vi "prep.vi"(8 "error in (no error)":errorcluster, 9 "Coordinate System":enum16{"Cartesian", "Cylindrical", "Spherical"}(ring), 10 "Plot processed data In":T1 caption="Data In", 11 "Parametric in":refnum<class "Parametric.lvclass">) -> (0 "error out":errorcluster, 2 "Plot Processed Data Out":T1 caption="Data Out", 3 "Parametric out":refnum<class "Parametric.lvclass">)   [LabVIEW 2020, in "Parametric.lvclass"]
uses:
  <vilib>/Native 3D Graph/classes/Parametric/Parametric.lvclass
  <vilib>/Native 3D Graph/xcontrol/Processed Data.ctl
  <vilib>/Native 3D Graph/typedefs/plot_rep_array.ctl
  <vilib>/Native 3D Graph/typedefs/plot_rep.ctl
  <vilib>/Native 3D Graph/typedefs/range_cluster.ctl
  <vilib>/Native 3D Graph/typedefs/min_max.ctl
  <vilib>/Native 3D Graph/typedefs/plot_rep_mesh_data.ctl
  <vilib>/Native 3D Graph/classes/Parametric/Parametric.lvclass/Parametric.ctl
  <vilib>/Analysis/coordinate.llb/3D Coordinate Conversion (Scalar).vi
  <vilib>/Native 3D Graph/classes/Base Datatype.lvclass
  <vilib>/Native 3D Graph/xcontrol/3DPC_SurfacePlot.xctl
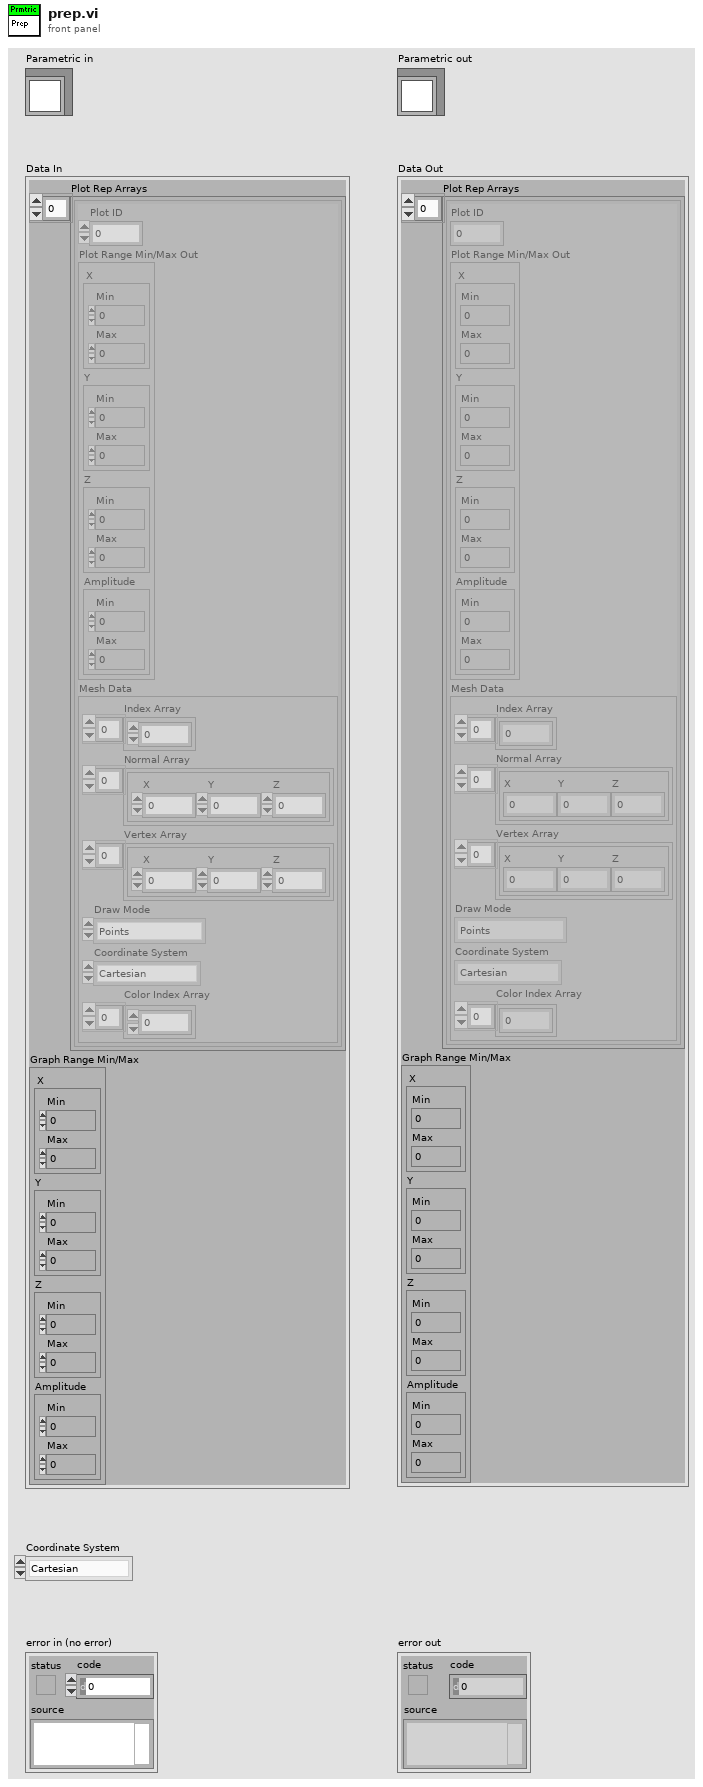
[diagram p1: front panel]
types:
  T1 = typedef "Processed Data.ctl" = cluster{"Plot Rep Arrays":T2, "Graph Range Min/Max":T4}
  T2 = typedef "3DPC_SurfacePlot.xctl/plot_rep_array.ctl" = T3[]
  T3 = typedef "3DPC_SurfacePlot.xctl/plot_rep.ctl" = cluster{"Plot ID":i32, "Plot Range Min/Max Out":T4, "Mesh Data":T6}
  T4 = typedef "3DPC_SurfacePlot.xctl/range_cluster.ctl" = cluster{"X":T5, "Y":T5, "Z":T5, "Amplitude":T5}
  T5 = typedef "3DPC_SurfacePlot.xctl/min_max.ctl" = cluster{"Min":sgl, "Max":sgl}
  T6 = typedef "3DPC_SurfacePlot.xctl/plot_rep_mesh_data.ctl" = cluster{"Index Array":u32[], "Normal Array":cluster{"X":sgl, "Y":sgl, "Z":sgl}[], "Vertex Array":cluster{"X":sgl, "Y":sgl, "Z":sgl}[], "Draw Mode":enum16{"Points", "Lines", "Line Strip", "Line Loop", "Triangles", "Triangle Strip", "Triangle Fan", "Quads", "Quad Strip", "Polygon"}, "Coordinate System":enum16{"Cartesian", "Cylindrical", "Spherical"}, "Color Index Array":i32[]}
  T7 = enum16{"Points", "Lines", "Line Strip", "Line Loop", "Triangles", "Triangle Strip", "Triangle Fan", "Quads", "Quad Strip", "Polygon"}
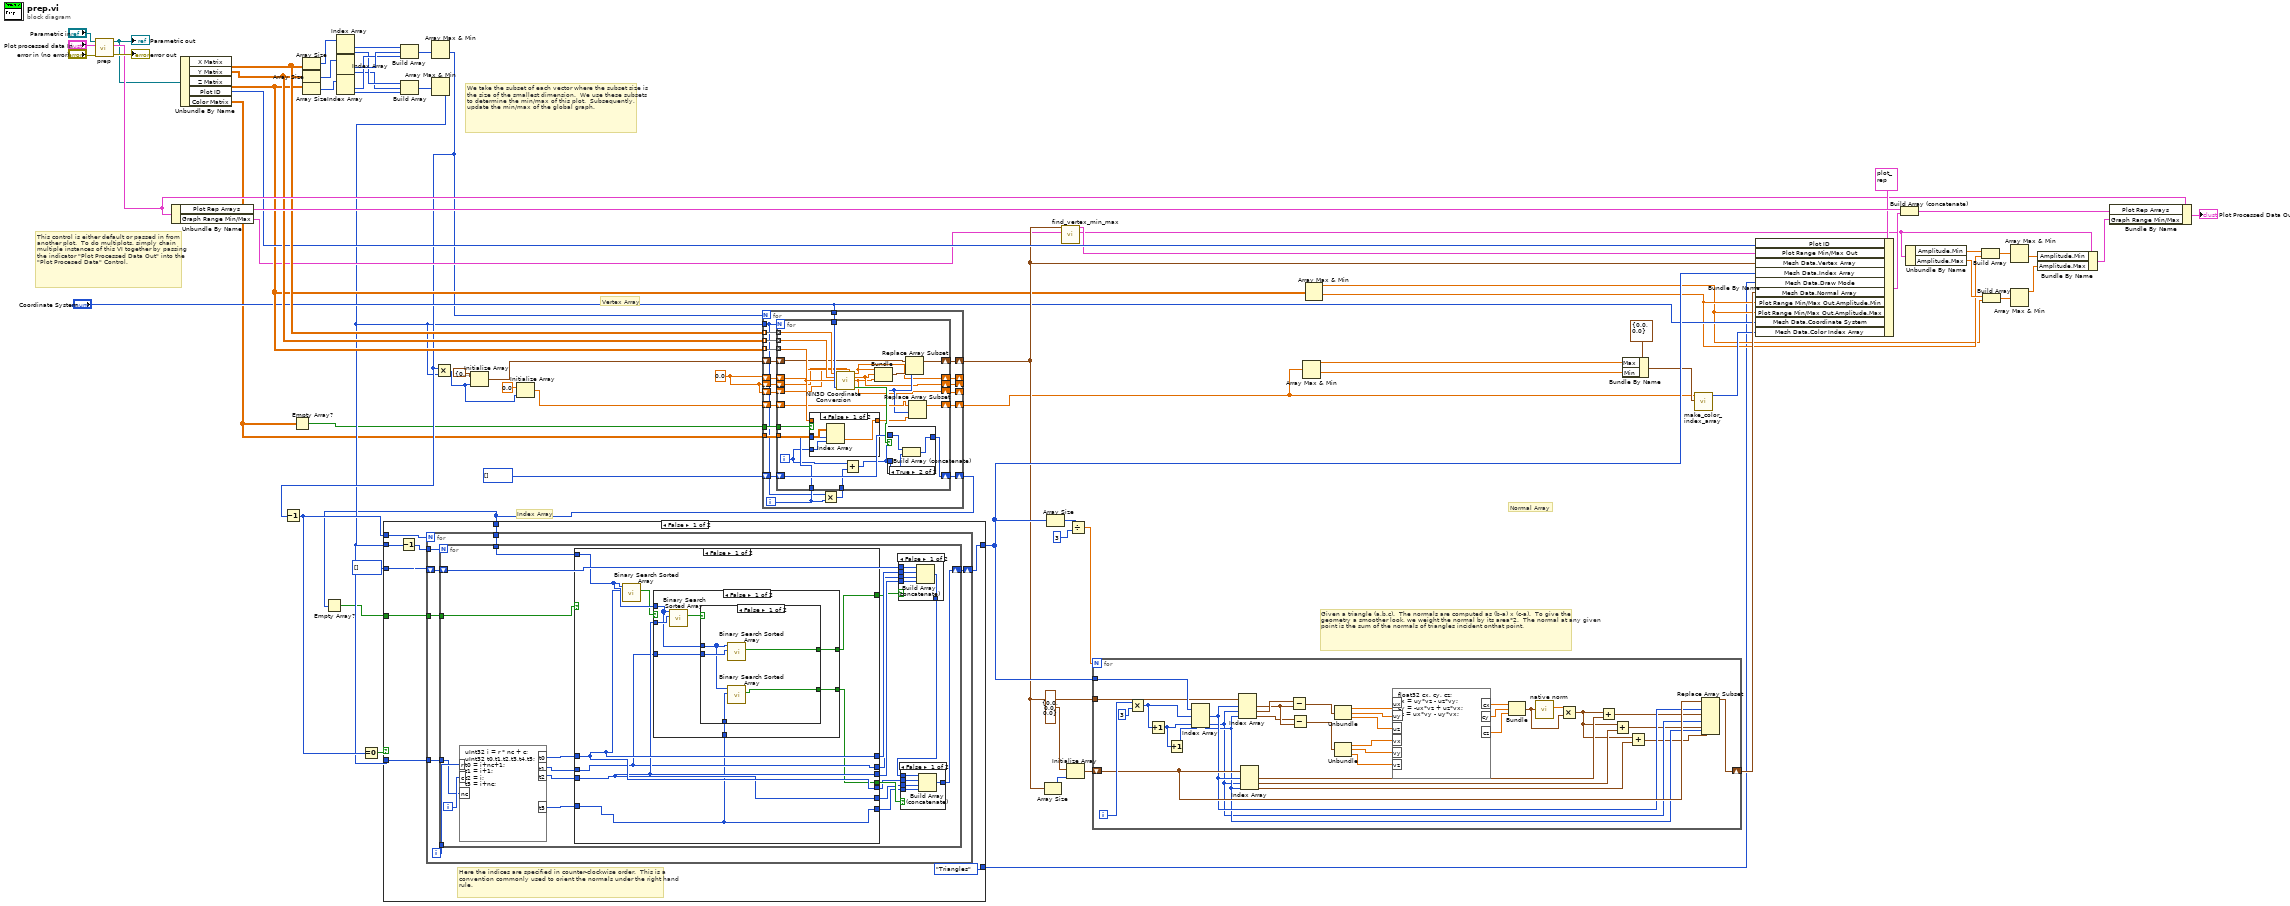
[diagram p0: block diagram]
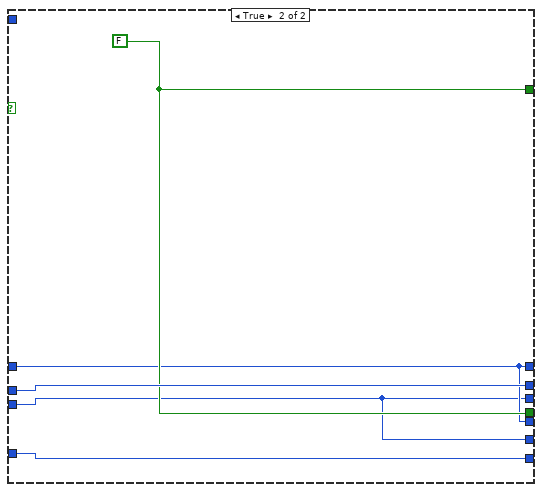
[diagram p6: hidden frame]
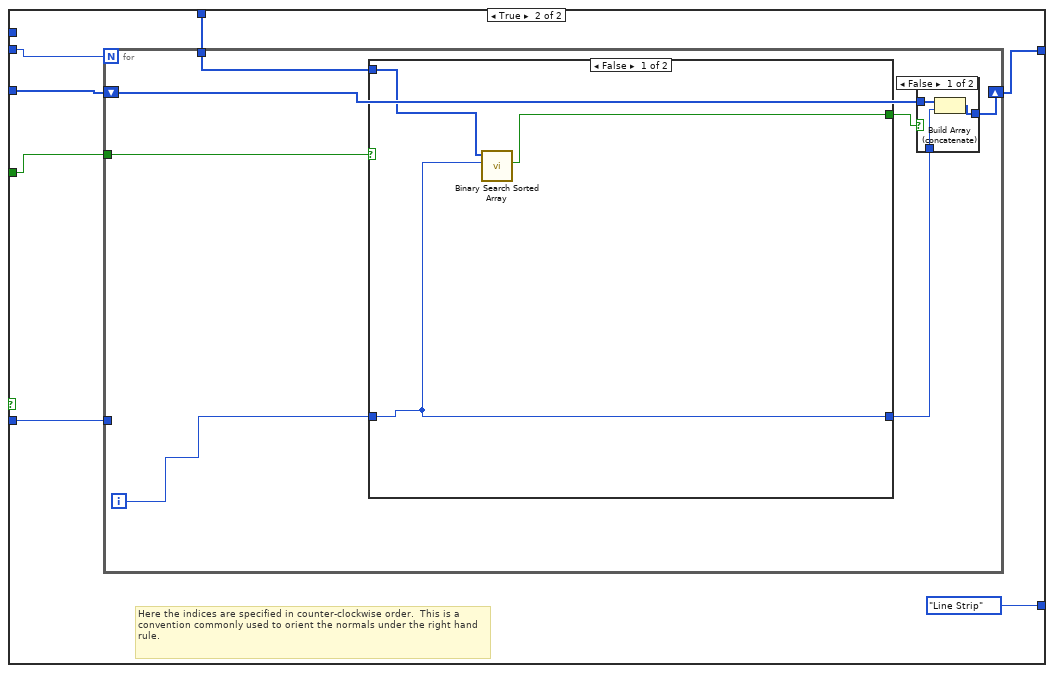
[diagram p7: hidden frame]
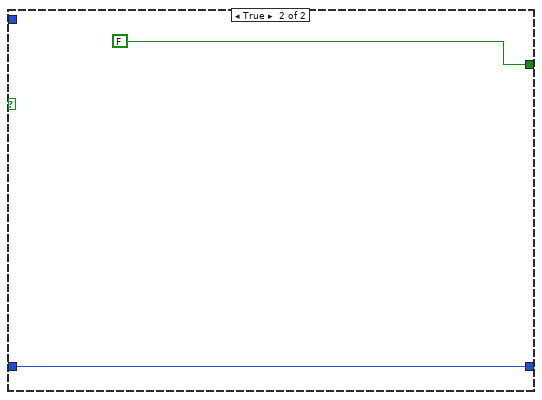
[diagram p9: hidden frame]
diagram:
  w7 = sgl 0.0
  # "Given a triangle (a,b,c).  The normals are computed as (b-a) x (c-a).  To give the geometry a smoother look, we weight the normal by its area*2.  The normal at any given point is the sum of the normals of triangles incident onthat point."
  # "Normal Array"
  # "Index Array"
  # "We take the subset of each vector where the subset size is the size of the smallest dimension.  We use these subsets to determine the min/max of this plot.  Subsequently, update the min/max of the global graph."
  # "This control is either default or passed in from another plot.  To do multiplots, simply chain multiple instances of this VI together by passing the indicator \"Plot Processed Data Out\" into the \"Plot Procesed Data\" Control."
  # "Vertex Array"
  n1 = call-parent "prep.vi"("error in (no error)"="error in (no error)", "Plot processed data In"="Plot processed data In", "Base Datatype in"="Parametric in") -> ("error out"=→"error out":errorcluster, "Plot processed Data Out"=w42:T1, "Base Datatype out"=w41:refnum<class "Parametric.lvclass">)  [unwired: 1 in, 5 out]
  "Parametric out" <- w41
  n2 = Unbundle By Name(w42) -> ("Plot Rep Arrays"=w66:T2, "Graph Range Min/Max"=w34:T4)
  n3 = Unbundle By Name(w41) -> ("X Matrix"=w40:sgl[][], "Y Matrix"=w39:sgl[][], "Z Matrix"=w35:sgl[][], "Plot ID"=w38:i32, "Color Matrix"=w4:sgl[][])
  n4 = Empty Array?(array=w4) -> (empty?=w3:bool)
  n5 = Array Size(array=w40) -> (size(s)=w62:i32[])
  n6 = Array Size(array=w39) -> (size(s)=w61:i32[])
  n7 = Array Size(array=w35) -> (size(s)=w60:i32[])
  n8 = Index Array(array=w62) -> (element #1=w59:i32, element #2=w56:i32)  [unwired: 2 in]
  n9 = Index Array(array=w61) -> (element #1=w58:i32, element #2=w55:i32)  [unwired: 2 in]
  n10 = Index Array(array=w60) -> (element #1=w57:i32, element #2=w54:i32)  [unwired: 2 in]
  n11 = Build Array(w59, w58, w57) -> (w53:i32[])
  n12 = Build Array(w56, w55, w54) -> (w52:i32[])
  n13 = Array Max & Min(array=w53) -> (min value=w14:i32)  [unwired: 3 out]
  n14 = Decrement(x=w14) -> (x-1=w17:i32)
  n15 = Equal To 0?(x=w17) -> (x = 0?=w16:bool)
  n16 = Array Max & Min(array=w52) -> (min value=w13:i32)  [unwired: 3 out]
  n17 = Multiply(x=w14, y=w13) -> (x*y=w9:i32)
  n18 = Initialize Array(cluster{"X":sgl, "Y":sgl, "Z":sgl} {"X"=0.0, "Y"=0.0, "Z"=0.0} ("3D Point"), w9) -> (w11:cluster{"X":sgl, "Y":sgl, "Z":sgl}[])
  n19 = Initialize Array(sgl 0.0, w9) -> (w8:sgl[])
  n20 = for {
    N: w14 -> [_]
    tunnel: w40 -> [w92] mode=indexing
    tunnel: w39 -> [w91] mode=indexing
    tunnel: w35 -> [w90] mode=indexing
    tunnel: w13 -> [w79]
    shift-right: [w88] -> w37
    shift-left: w11 -> [w89]
    tunnel: "Coordinate System" -> [w87]
    shift-right: [w85] -> w20
    shift-left: w8 -> [w86]
    tunnel: w3 -> [w84]
    tunnel: w4 -> [w83]
    shift-right: [w81] -> w6
    shift-left: u32[] [] -> [w82]
    shift-right: [w74] -> _
    shift-left: w7 -> [w77]
    shift-right: [w73] -> _
    shift-left: w7 -> [w76]
    shift-right: [w72] -> _
    shift-left: w7 -> [w75]
    i -> [w80]
    n21 = Multiply(x=w79, y=w80) -> (x*y=w78:i32)
    n22 = for {
      N: w79 -> [_]
      shift-right: [w104] -> w88
      shift-left: w89 -> [w105]
      tunnel: w92 -> [w115] mode=indexing
      tunnel: w91 -> [w116] mode=indexing
      tunnel: w90 -> [w113] mode=indexing
      tunnel: w87 -> [w117]
      shift-right: [w101] -> w85
      shift-left: w86 -> [w102]
      tunnel: w84 -> [w114]
      tunnel: w83 -> [w112]
      tunnel: w80 -> [w108]
      shift-right: [w109] -> w81
      shift-left: w82 -> [w110]
      tunnel: w78 -> [w107]
      shift-right: [w95] -> w74
      shift-left: w77 -> [w98]
      shift-right: [w94] -> w73
      shift-left: w76 -> [w97]
      shift-right: [w93] -> w72
      shift-left: w75 -> [w96]
      i -> [w106]
      n23 = case shown="False" w114 {
        tunnel: w113 -> [_ w126]
        tunnel: [w122 w126] -> w99
        tunnel: w112 -> [w125 _]
        tunnel: w108 -> [w124 _]
        tunnel: w106 -> [w123 _]
        frame False {
          n24 = Index Array(array=w125, index (row)=w124, index (col)=w123) -> (element=w122:sgl)
        }
        frame True {
        }
      }
      n25 = call <vilib>:"NIN3D Coordinate Conversion.vi"("X"=w115, "Z_prev"=w96, "Y_prev"=w97, "X_prev"=w98, "Y"=w116, "Z"=w113, "Coordinate System"=w117) -> ("X out"=w95:sgl, "Y out"=w94:sgl, "Z out"=w93:sgl, "NaN?"=w111:bool)  [unwired: 5 in]
      n26 = Add(x=w106, y=w107) -> (x+y=w100:i32)
      n27 = Bundle("X out"=w95, "Y out"=w94, "Z out"=w93) -> (w103:cluster{"X out":sgl, "Y out":sgl, "Z out":sgl})  [unwired: 1 out]
      n28 = case shown="True" w111 {
        tunnel: w110 -> [w118 w121]
        tunnel: [w118 w120] -> w109
        tunnel: w100 -> [_ w119]
        frame False {
        }
        frame True {
          n29 = Build Array (concatenate)(w121, w119) -> (w120:u32[])
        }
      }
      n30 = Replace Array Subset(array=w105, new element=w103, index=w100) -> (w104:cluster{"X":sgl, "Y":sgl, "Z":sgl}[])
      n31 = Replace Array Subset(array=w102, new element=w99, index=w100) -> (w101:sgl[])
    }
  }
  n32 = Empty Array?(array=w6) -> (empty?=w5:bool)
  n33 = case shown="False" w16 {
    tunnel: u32[] [] ("Indices") -> [w127 w208]
    tunnel: w13 -> [w135 w207]
    tunnel: [w134 w206] -> w44
    tunnel: w17 -> [w133 _]
    tunnel: w6 -> [w132 w205]
    tunnel: w13 -> [w131 w204]
    tunnel: [T7."Triangles" ("Mesh Data.Draw Mode") T7."Line Strip" ("Mesh Data.Draw Mode")] -> w2
    tunnel: w5 -> [w128 w202]
    frame False {
      # "Here the indices are specified in counter-clockwise order.  This is a convention commonly used to orient the normals under the right hand rule."
      n34 = Decrement(x=w131) -> (x-1=w130:i32)
      n35 = for {
        N: w133 -> [_]
        shift-right: [w138] -> w134
        shift-left: w127 -> [w142]
        tunnel: w130 -> [w140]
        tunnel: w135 -> [w139]
        tunnel: w132 -> [w137]
        tunnel: w128 -> [w136]
        i -> [w141]
        n36 = for {
          N: w140 -> [_]
          tunnel: w141 -> [w161]
          tunnel: w139 -> [w159]
          shift-right: [w147] -> w138
          shift-left: w142 -> [w162]
          tunnel: w137 -> [w154]
          tunnel: w136 -> [w143]
          i -> [w160]
          n37 = formula code="uInt32 i = r * nc + c; \nuInt32 t0,t1,t2,t3,t4,t5;\nt0 = i+nc+1; \nt1 = i+1; \nt2 = i; \nt5 = i+nc;"("r"=w161, "nc"=w159, "c"=w160) -> ("t0"=w158:u32, "t1"=w157:u32, "t2"=w156:u32, "t5"=w155:u32)
          n38 = case shown="False" w143 {
            tunnel: w154 -> [w182 _]
            tunnel: w158 -> [w181 w198]
            tunnel: [w181 w198] -> w153
            tunnel: w157 -> [w177 w201]
            tunnel: [w177 w201] -> w152
            tunnel: w156 -> [w178 w197]
            tunnel: [w178 w197] -> w151
            tunnel: [w181 w198] -> w146
            tunnel: [w178 w197] -> w145
            tunnel: w155 -> [w176 w200]
            tunnel: [w176 w200] -> w144
            tunnel: [w180 w199] -> w150
            tunnel: [w175 w199] -> w149
            frame False {
              n39 = call <vilib>:"Binary Search Sorted Array.vi"("Element"=w181, "Sorted Array"=w182) -> ("Found?"=w179:bool)  [unwired: 9 in]
              n40 = case shown="False" w179 {
                selector: w179 -> [_ w196]
                tunnel: w182 -> [w187 _]
                tunnel: w178 -> [w189 _]
                tunnel: [w186 w196] -> w180
                tunnel: w177 -> [w185 _]
                tunnel: w176 -> [w184 _]
                tunnel: [w183 w196] -> w175
                frame False {
                  n41 = call <vilib>:"Binary Search Sorted Array.vi"("Element"=w189, "Sorted Array"=w187) -> ("Found?"=w188:bool)  [unwired: 9 in]
                  n42 = case shown="False" w188 {
                    selector: w188 -> [_ w195]
                    tunnel: w187 -> [w191 _]
                    tunnel: w185 -> [w194 _]
                    tunnel: [w193 w195] -> w186
                    tunnel: w184 -> [w192 _]
                    tunnel: [w190 w195] -> w183
                    frame False {
                      n43 = call <vilib>:"Binary Search Sorted Array.vi"("Element"=w194, "Sorted Array"=w191) -> ("Found?"=w193:bool)  [unwired: 9 in]
                      n44 = call <vilib>:"Binary Search Sorted Array.vi"("Element"=w192, "Sorted Array"=w191) -> ("Found?"=w190:bool)  [unwired: 9 in]
                    }
                    frame True {
                    }
                  }
                }
                frame True {
                }
              }
            }
            frame True {
              w199 = FALSE
            }
          }
          n45 = case shown="False" w150 {
            tunnel: w162 -> [w173 w174]
            tunnel: w153 -> [w172 _]
            tunnel: w152 -> [w171 _]
            tunnel: w151 -> [w170 _]
            tunnel: [w169 w174] -> w148
            frame False {
              n46 = Build Array (concatenate)(w173, w172, w171, w170) -> (w169:u32[])
            }
            frame True {
            }
          }
          n47 = case shown="False" w149 {
            tunnel: w148 -> [w167 w168]
            tunnel: [w166 w168] -> w147
            tunnel: w146 -> [w165 _]
            tunnel: w145 -> [w164 _]
            tunnel: w144 -> [w163 _]
            frame False {
              n48 = Build Array (concatenate)(w167, w165, w164, w163) -> (w166:u32[])
            }
            frame True {
            }
          }
        }
      }
    }
    frame True {
      # "Here the indices are specified in counter-clockwise order.  This is a convention commonly used to orient the normals under the right hand rule."
      n49 = for {
        N: w204 -> [_]
        tunnel: w207 -> [_]
        shift-right: [w214] -> w206
        shift-left: w208 -> [w215]
        tunnel: w205 -> [w213]
        tunnel: w202 -> [w209]
        i -> [w210]
        n50 = case shown="False" w209 {
          tunnel: w213 -> [w222 _]
          tunnel: w210 -> [w221 w223]
          tunnel: [w220 FALSE] -> w212
          tunnel: [w221 w223] -> w211
          frame False {
            n51 = call <vilib>:"Binary Search Sorted Array.vi"("Element"=w221, "Sorted Array"=w222) -> ("Found?"=w220:bool)  [unwired: 9 in]
          }
          frame True {
          }
        }
        n52 = case shown="False" w212 {
          tunnel: w215 -> [w218 w219]
          tunnel: [w217 w219] -> w214
          tunnel: w211 -> [w216 _]
          frame False {
            n53 = Build Array (concatenate)(w218, w216) -> (w217:u32[])
          }
          frame True {
          }
        }
      }
    }
  }
  n54 = Array Size(array=w37) -> (size(s)=w50:i32)
  n55 = Array Size(array=w44) -> (size(s)=w46:i32)
  n56 = call <vilib>:"find_vertex_min_max.vi"("Total Range Min/Max"=w34, "Vertex Array"=w37) -> ("Total Range Out"=w25:T4, "This Range Min/Max Out"=w36:T4)  [unwired: 8 out]
  n57 = Initialize Array(cluster{"X":sgl, "Y":sgl, "Z":sgl} {"X"=0.0, "Y"=0.0, "Z"=0.0} ("3D Point"), w50) -> (w49:cluster{"X":sgl, "Y":sgl, "Z":sgl}[])
  n58 = Divide(x=w46, y=3) -> (x/y=w47:dbl)
  n59 = for {
    N: w47 -> [_]
    shift-right: [w251] -> w43
    shift-left: w49 -> [w254]
    tunnel: w44 -> [w257]
    tunnel: w37 -> [w249]
    i -> [w259]
    n60 = Multiply(x=w259, y=3) -> (x*y=w256:i32)
    n61 = Increment(x=w256) -> (x+1=w250:i32)
    n62 = Increment(x=w250) -> (x+1=w255:i32)
    n63 = Index Array(array=w257, index #1=w256, index #2=w250, index #3=w255) -> (element #1=w253:u32, element #2=w248:u32, element #3=w252:u32)
    n64 = Index Array(array=w249, index #1=w253, index #2=w248, index #3=w252) -> (element #1=w246:cluster{"X":sgl, "Y":sgl, "Z":sgl}, element #2=w247:cluster{"X":sgl, "Y":sgl, "Z":sgl}, element #3=w239:cluster{"X":sgl, "Y":sgl, "Z":sgl})
    n65 = Index Array(array=w254, index #1=w253, index #2=w248, index #3=w252) -> (element #1=w245:cluster{"X":sgl, "Y":sgl, "Z":sgl}, element #2=w244:cluster{"X":sgl, "Y":sgl, "Z":sgl}, element #3=w242:cluster{"X":sgl, "Y":sgl, "Z":sgl})
    n66 = Subtract(x=w247, y=w246) -> (x-y=w227:cluster{"X":sgl, "Y":sgl, "Z":sgl})
    n67 = Subtract(x=w239, y=w246) -> (x-y=w226:cluster{"X":sgl, "Y":sgl, "Z":sgl})
    n68 = Unbundle(w227) -> ("X"=w236:sgl, "Y"=w235:sgl, "Z"=w234:sgl)
    n69 = Unbundle(w226) -> ("X"=w233:sgl, "Y"=w232:sgl, "Z"=w231:sgl)
    n70 = formula code="float32 cx, cy, cz;\ncx = uy*vz - uz*vy;\ncy = -ux*vz + uz*vx;\ncz = ux*vy - uy*vx;"("ux"=w236, "uy"=w235, "uz"=w234, "vx"=w233, "vy"=w232, "vz"=w231) -> ("cx"=w230:sgl, "cy"=w229:sgl, "cz"=w228:sgl)
    n71 = Bundle(w230, w229, w228) -> (w225:cluster{sgl, sgl, sgl})  [unwired: 1 out]
    n72 = call <vilib>:"native norm.vi"("Vector"=w225) -> ("Norm"=w237:sgl)  [unwired: 10 in]
    n73 = Multiply(x=w237, y=w225) -> (x*y=w243:cluster{sgl, sgl, sgl})
    n74 = Add(x=w243, y=w245) -> (x+y=w238:cluster{sgl, sgl, sgl})
    n75 = Add(x=w243, y=w244) -> (x+y=w241:cluster{sgl, sgl, sgl})
    n76 = Add(x=w243, y=w242) -> (x+y=w240:cluster{sgl, sgl, sgl})
    n77 = Replace Array Subset(array=w254, new element #1=w238, index #1=w253, new element #2=w241, index #2=w248, new element #3=w240, index #3=w252) -> (w251:cluster{"X":sgl, "Y":sgl, "Z":sgl}[])
  }
  n78 = Array Max & Min(array=w20) -> (max value=w18:sgl, min value=w1:sgl)  [unwired: 2 out]
  n79 = Array Max & Min(array=w35) -> (max value=w19:sgl, min value=w21:sgl)  [unwired: 2 out]
  n80 = Bundle By Name(cluster=T5 {"Min"=0.0, "Max"=0.0} ("Amplitude"), "Max"=w18, "Min"=w1) -> (w23:T5)
  n81 = call <vilib>:"make_color_index_array.vi"("Amplitude Min/Max"=w23, "Z array"=w20) -> ("Color Index Array"=w22:i32[])  [unwired: 9 out]
  n82 = Bundle By Name(cluster=T3 {"Plot ID"=0, "Plot Range Min/Max Out"={"X"={"Min"=0.0, "Max"=0.0}, "Y"={"Min"=0.0, "Max"=0.0}, "Z"={"Min"=0.0, "Max"=0.0}, "Amplitude"={"Min"=0.0, "Max"=0.0}}, "Mesh Data"={"Index Array"=[], "Normal Array"=[], "Vertex Array"=[], "Draw Mode"=enum."Points", "Coordinate System"=enum."Cartesian", "Color Index Array"=[]}} ("Plot Representation"), "Plot ID"=w38, "Plot Range Min/Max Out"=w36, "Mesh Data.Vertex Array"=w37, "Mesh Data.Index Array"=w44, "Mesh Data.Draw Mode"=w2, "Mesh Data.Normal Array"=w43, "Plot Range Min/Max Out.Amplitude.Min"=w21, "Plot Range Min/Max Out.Amplitude.Max"=w19, "Mesh Data.Coordinate System"="Coordinate System", "Mesh Data.Color Index Array"=w22) -> (w65:T3)
  n83 = Build Array (concatenate)(w66, w65) -> (w64:T2)
  n84 = Unbundle By Name(w25) -> ("Amplitude.Min"=w32:sgl, "Amplitude.Max"=w29:sgl)
  n85 = Build Array(w32, w21) -> (w31:sgl[])
  n86 = Build Array(w29, w19) -> (w28:sgl[])
  n87 = Array Max & Min(array=w31) -> (min value=w30:sgl)  [unwired: 3 out]
  n88 = Array Max & Min(array=w28) -> (max value=w27:sgl)  [unwired: 3 out]
  n89 = Bundle By Name(cluster=w25, "Amplitude.Min"=w30, "Amplitude.Max"=w27) -> (w26:T4)
  n90 = Bundle By Name(cluster=w42, "Plot Rep Arrays"=w64, "Graph Range Min/Max"=w26) -> (→"Plot Processed Data Out":T1)
